vi "Workspace.Select.Dialog.vi"(10 "CD Path":string, 11 "NIVS.System Definition Root":refnum<k24>) -> (1 "Cancelled?":bool, 2 "IP Address":string="Targets/Controller/Custom Devices/Communication Example", 3 "Custom Device Path Out":string="Targets/Controller/Custom Devices/Communication Example")   [LabVIEW 2015, in "Diagnostics Addon Shared.lvlib"]
uses:
  Diagnostics Addon Shared.lvlib
  NationalInstruments.VeriStand.SystemStorage
panel:
  in  "Cancel":bool
  in  "Select":bool
  in  "Custom Device Path":string(tree)
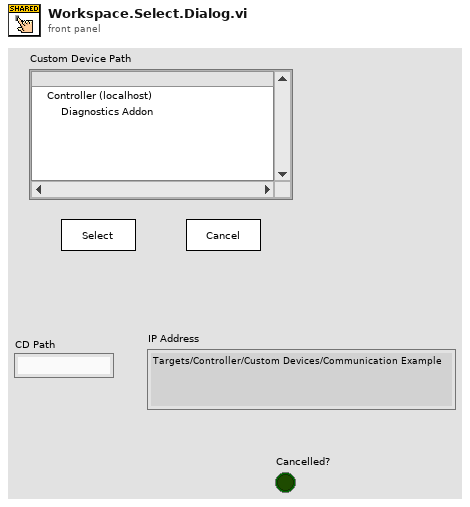
[diagram p1: front panel]
types:
  T1 = enum8{"Enabled", "Disabled", "Disabled and Grayed Out"}
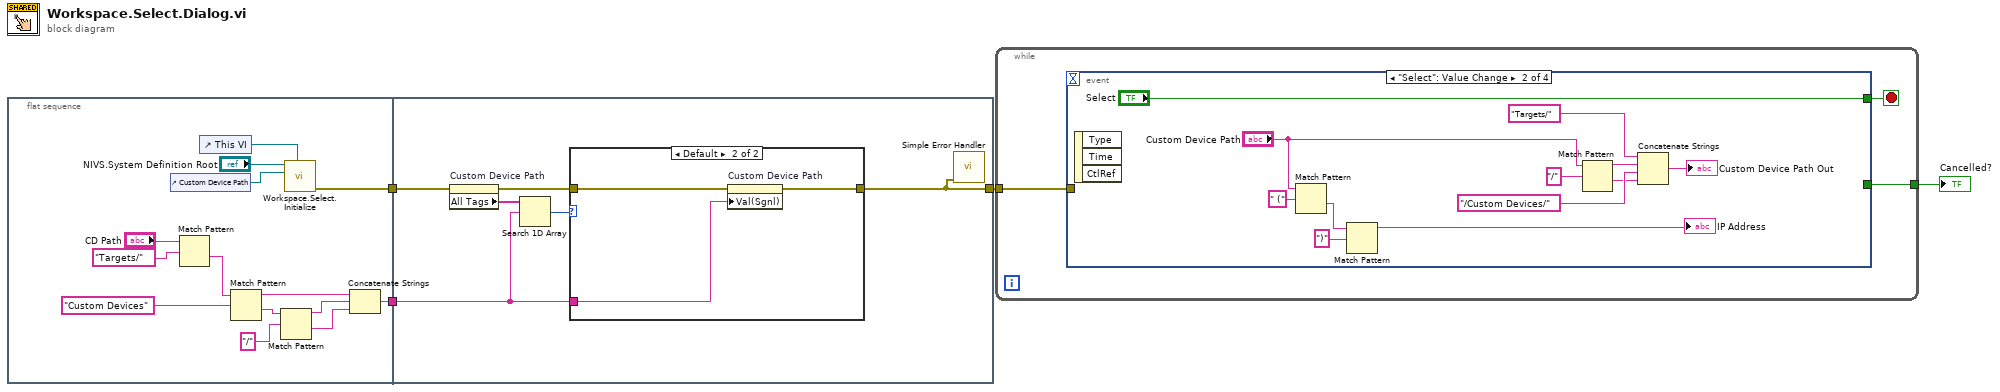
[diagram p0: block diagram]
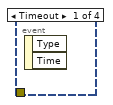
[diagram p2: hidden frame]
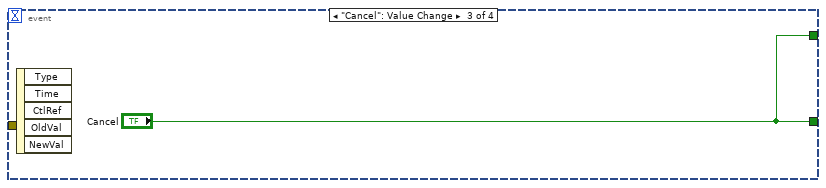
[diagram p3: hidden frame]
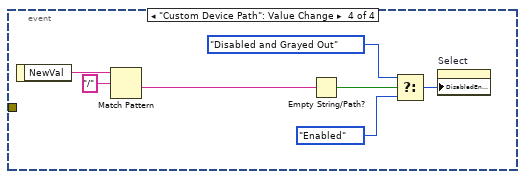
[diagram p4: hidden frame]
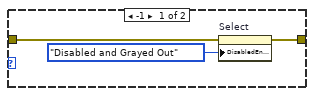
[diagram p5: hidden frame]
diagram:
  n1 = flat-sequence {
    tunnel: [w16] -> w3
    tunnel: [w9] -> w1
    tunnel: [w24] -> w4
    tunnel: w3 -> [w23]
    tunnel: w1 -> [w20]
    frame #0 {
      n2 = control-ref of="Custom Device Path"() -> (w17:refnum<vi>)
      n3 = Match Pattern(string="CD Path", regular expression="Targets/") -> (after substring=w12:string)  [unwired: 1 in, 3 out]
      n4 = control-ref of="This VI"() -> (w15:refnum<vi>)
      n5 = Match Pattern(string=w12, regular expression="Custom Devices") -> (before substring=w14:string, after substring=w8:string)  [unwired: 1 in, 2 out]
      n6 = Match Pattern(string=w8, regular expression="/") -> (before substring=w6:string, after substring=w5:string)  [unwired: 1 in, 2 out]
      n7 = call "Workspace.Select.Initialize.vi"("VI reference (current VI)"=w15, "Tree"=w17, "NIVS.System Definition Root"="NIVS.System Definition Root") -> ("error out"=w16:errorcluster)  [unwired: 7 in, 1 out]
      n8 = Concatenate Strings(w14, w6, w5) -> (w9:string)
    }
    frame #1 {
      n9 = property on="Custom Device Path" class="Tree (strict)"(error in=w23) -> (error out=w22:errorcluster, "All Tags"=w21:string[])  [unwired: 1 in, 1 out]
      n10 = Search 1D Array(1D array=w21, element=w20) -> (index of element=w19:i32)  [unwired: 1 in]
      n11 = case shown="Default" w19 {
        tunnel: [w27 w30] -> w24
        tunnel: w22 -> [w26 w29]
        tunnel: w20 -> [_ w28]
        frame -1 {
          n12 = property on="Select" class="Bool"(error in=w26, "DisabledEnum"=T1."Disabled and Grayed Out" ("Disabled")) -> (error out=w27:errorcluster)  [unwired: 1 in, 1 out]
        }
        frame Default {
          n13 = property on="Custom Device Path" class="Tree (strict)"(error in=w29, "Val(Sgnl)"=w28) -> (error out=w30:errorcluster)  [unwired: 1 in, 1 out]
        }
      }
      n14 = call <vilib>:"Simple Error Handler.vi"("error in (no error)"=w24) -> ()  [unwired: 4 in, 5 out]
    }
  }
  n15 = while {
    tunnel: w4 -> [w33]
    tunnel: [w31] -> w2
    stop <- w32 stop-if-true
    n16 = event shown="[1] \"Select\": Value Change" {
      selector: _ -> [_ _ _ _]
      dyn-events: _ -> [_ _ _ _]
      timeout: _ -> [_ _ _ _]
      tunnel: w33 -> [_ _ _ _]
      tunnel: [_ "Select" "Cancel" _] -> w32
      tunnel: [_ _ "Cancel" _] -> w31
      event Timeout {
        n17 = event-data() -> ()  [unwired: 1 in, 2 out]
      }
      event "Select": Value Change {
        n18 = event-data() -> ()  [unwired: 1 in, 3 out]
        n19 = Match Pattern(string="Custom Device Path", regular expression=" (") -> (after substring=w36:string)  [unwired: 1 in, 3 out]
        n20 = Match Pattern(string=w36, regular expression=")") -> (before substring=→"IP Address":string)  [unwired: 1 in, 3 out]
        n21 = Match Pattern(string="Custom Device Path", regular expression="/") -> (before substring=w43:string, after substring=w41:string)  [unwired: 1 in, 2 out]
        n22 = Concatenate Strings("Targets/" ("string"), w43, "/Custom Devices/" ("string"), w41) -> (→"Custom Device Path Out":string)
      }
      event "Cancel": Value Change {
        n23 = event-data() -> ()  [unwired: 1 in, 5 out]
      }
      event "Custom Device Path": Value Change {
        n24 = event-data() -> ("NewVal"=w53:string)  [unwired: 1 in]
        n25 = Match Pattern(string=w53, regular expression="/") -> (after substring=w47:string)  [unwired: 1 in, 3 out]
        n26 = Empty String/Path?(string/path=w47) -> (empty?=w52:bool)
        n27 = Select(t=T1."Disabled and Grayed Out" ("Disabled"), s=w52, f=T1."Enabled" ("Disabled")) -> (s? t:f=w49:T1)
        n28 = property on="Select" class="Bool"("DisabledEnum"=w49) -> ()  [unwired: 2 in, 2 out]
      }
    }
  }
  "Cancelled?" <- w2
